vi "Sort by muon hit time.vi"(2 "Top Coincs saving":T2, 3 "Type":enum16{"internal", "saving"}(ring)=enum."saving", 4 "Top Coincs internal":T1[](array[typedef])) -> (0 "Coincidences saving":T2, 1 "Coincidences internal":T1[](array[typedef]))   [LabVIEW 2016]
uses:
  Typedefs/CoincidencesToSave.ctl
  Typedefs/CoincidenceWithGPSformat.ctl
  Typedefs/Coincidence.ctl
  Global Variables/System info.vi
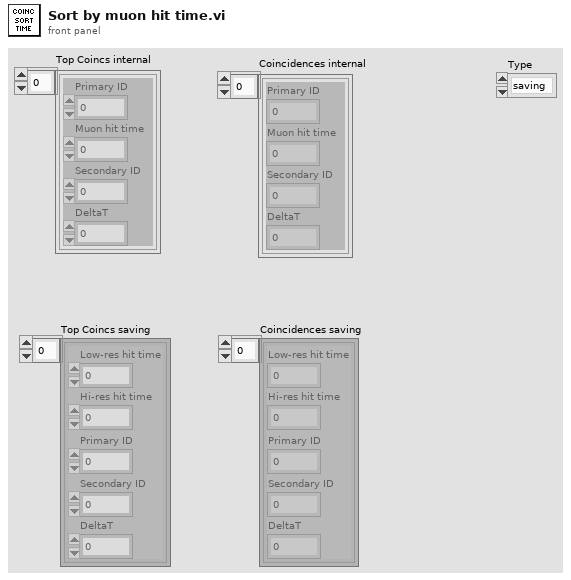
[diagram p1: front panel]
types:
  T1 = typedef "Coincidence.ctl" = cluster{"Primary ID":i8, "Muon hit time":u64, "Secondary ID":i8, "DeltaT":i32}
  T2 = typedef "CoincidencesToSave.ctl" = T3[]
  T3 = typedef "CoincidenceWithGPSformat.ctl" = cluster{"Low-res hit time":u32, "Hi-res hit time":u32, "Secondary ID":i8, "DeltaT":i32, "Primary ID":i8}
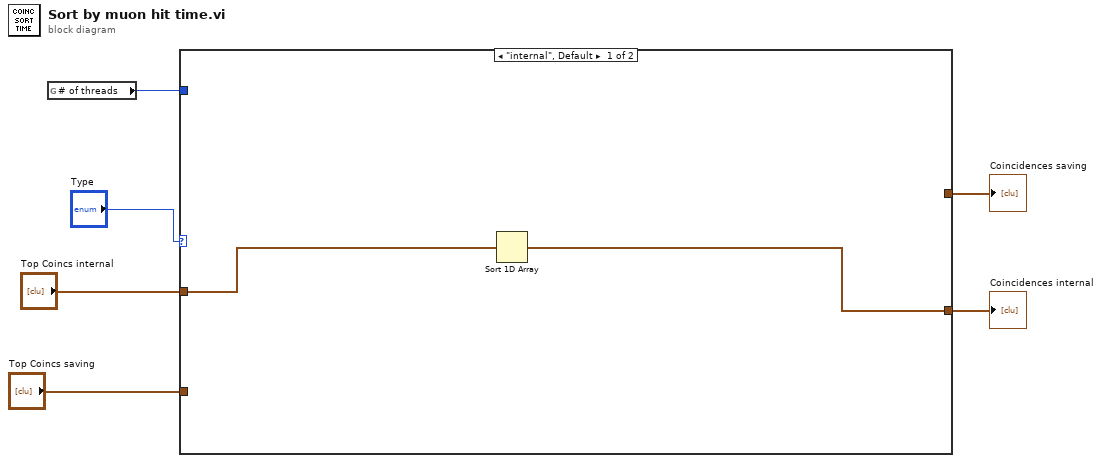
[diagram p0: block diagram]
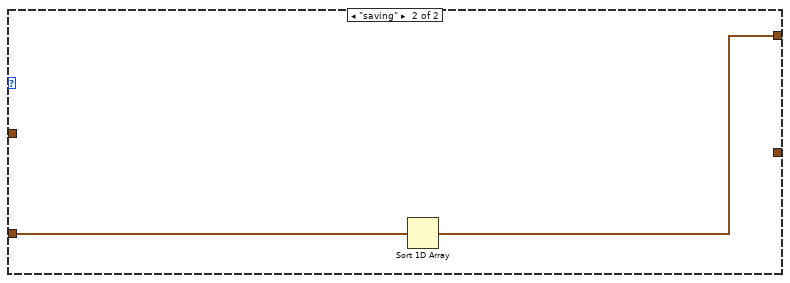
[diagram p2: hidden frame]
diagram:
  n1 = global read "System info.vi" "# of threads"() -> (w5:i32)
  n2 = case shown="\"internal\", Default" "Type" {
    tunnel: [_ w9] -> w6
    tunnel: "Top Coincs saving" -> [_ w10]
    tunnel: w5 -> [_ _]
    tunnel: "Top Coincs internal" -> [w8 _]
    tunnel: [w7 _] -> w1
    frame "internal", Default {
      n3 = Sort 1D Array(array=w8) -> (sorted array=w7:T1[])
    }
    frame "saving" {
      n4 = Sort 1D Array(array=w10) -> (sorted array=w9:T2)
    }
  }
  "Coincidences saving" <- w6
  "Coincidences internal" <- w1
